vi "Current Max Read Array.vi"(8 "error in":errorcluster, 11 "Cycler in":refnum<class "Cycler.lvclass">) -> (0 "error out":errorcluster, 1 "Changed or First Call?":bool, 2 "Current Max SP":dbl[](array[numeric]), 3 "Cycler out":refnum<class "Cycler.lvclass">)   [LabVIEW 2023, in "Cycler.lvclass"]
uses:
  Cycler.lvclass
  Low Level Capabilities/Current/Current Limit/Current Limit.lvclass
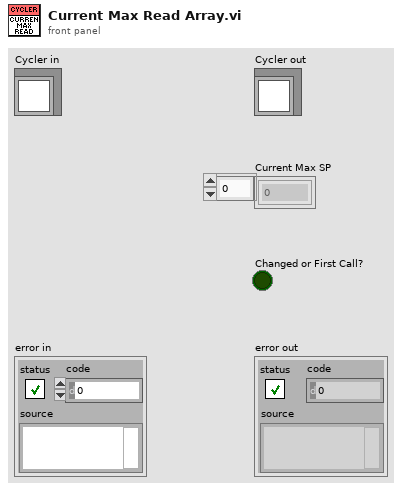
[diagram p1: front panel]
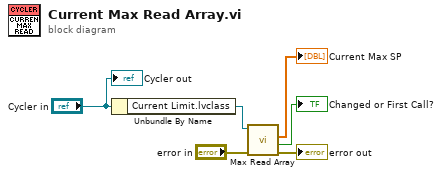
[diagram p0: block diagram]
diagram:
  n1 = Unbundle By Name("Cycler in") -> ("Current Limit.lvclass"=w6:refnum<class "Current Limit.lvclass">)
  n2 = call-dynamic "Max Read Array.vi"("error in"="error in", "Max Current Limit in"=w6) -> ("error out"=→"error out":errorcluster, "Changed or First Call?"=→"Changed or First Call?":bool, "Current Max SP"=→"Current Max SP":dbl[])  [unwired: 6 in, 1 out]
  "Cycler out" <- "Cycler in"
